vi "Test.vi"() -> ()   [LabVIEW 2018]
uses:
  utils/Return_t.ctl
  <vilib>/Instr/_visa.llb/VISA Configure Serial Port (Instr).vi
panel:
  out "Read DATA Str":string
  out "Str EPC":string
  out "EPC Bytes":u8
  out "Freq (Mhz)":dbl
  out "RSSI":i32
  out "Return":T1
  out "Shift Data":u16
  out "Msg Length":u16
  out "FF?":bool
  in  "stop":bool
  in  "Test":bool
  in  "Power":u32=500 max=2700 step=10
  out "error out":errorcluster
  out "Read DATA HEX":string
  in  "Delay":u16=1200
  out "Set Err":errorcluster
  out "WR Str":string
  out "Ini ?":bool
  in  "COM RFID":refnum<visa-resource-name>="COM4"
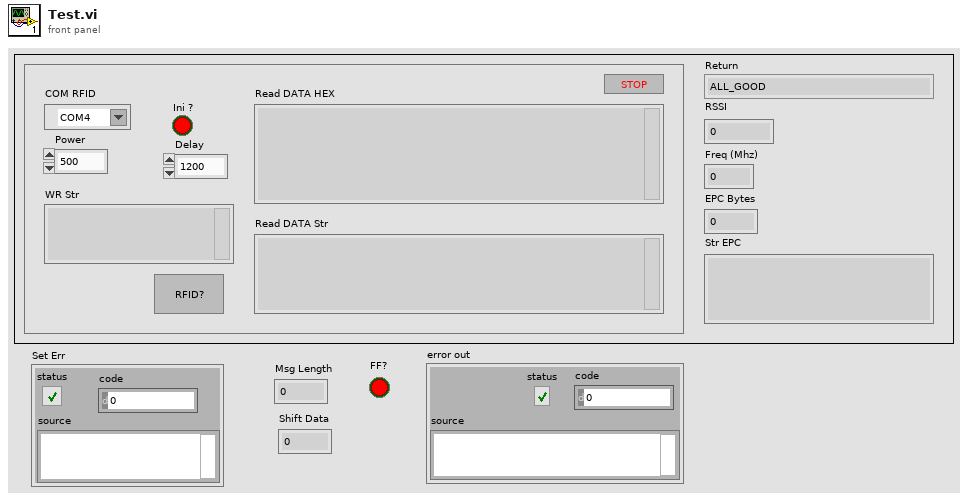
[diagram p1: front panel]
types:
  T1 = typedef "Return_t.ctl" = enum16{"ALL_GOOD", "ERROR_COMMAND_RESPONSE_TIMEOUT", "ERROR_CORRUPT_RESPONSE", "ERROR_WRONG_OPCODE_RESPONSE", "ERROR_UNKNOWN_OPCODE", "RESPONSE_IS_TEMPERATURE", "RESPONSE_IS_KEEPALIVE", "RESPONSE_IS_TEMPTHROTTLE", "RESPONSE_IS_TAGFOUND", "RESPONSE_IS_NOTAGFOUND", "RESPONSE_IS_UNKNOWN", "RESPONSE_SUCCESS", "RESPONSE_FAIL"}
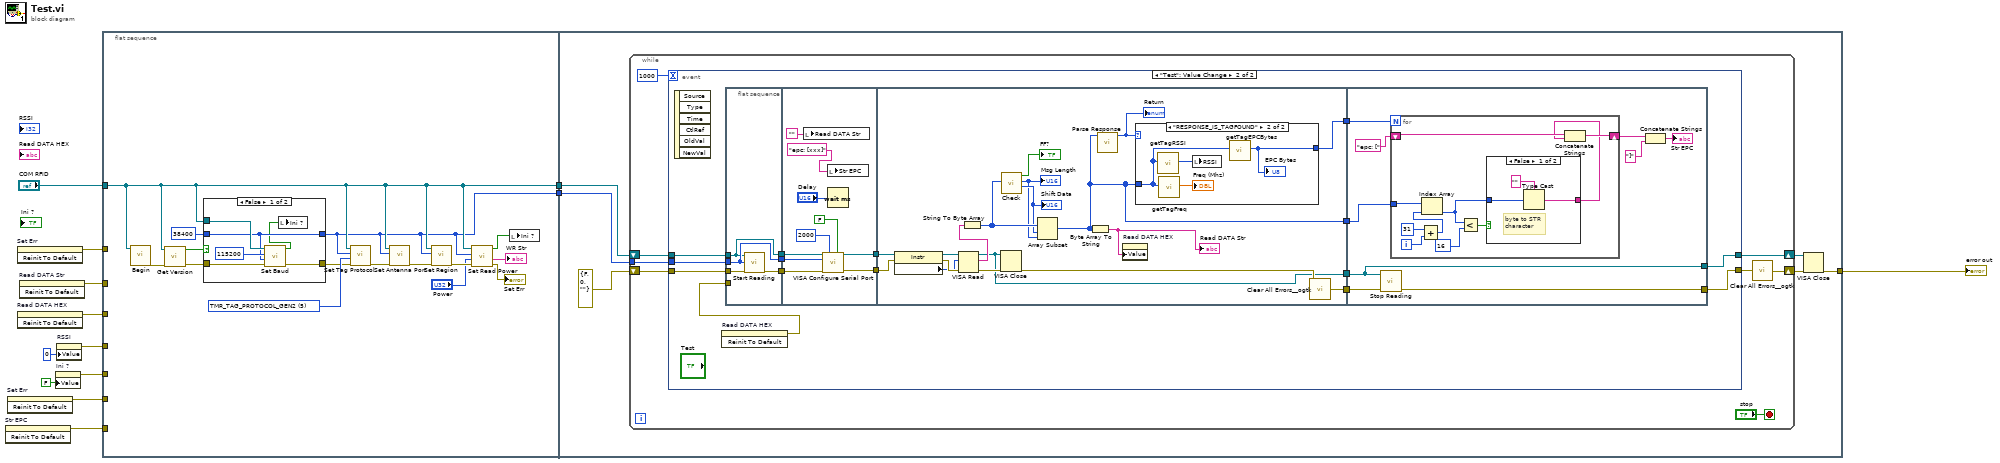
[diagram p0: block diagram]
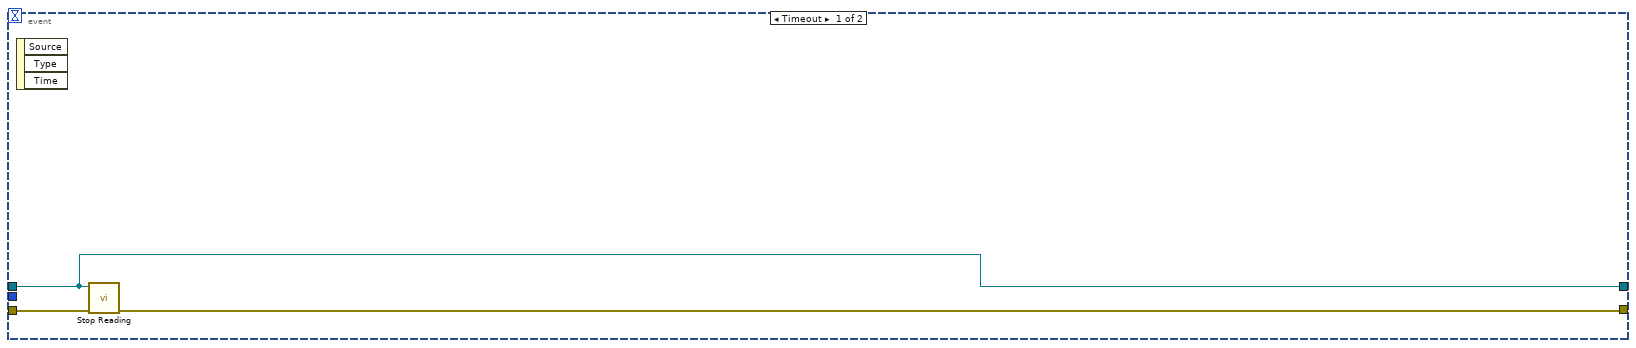
[diagram p3: hidden frame]
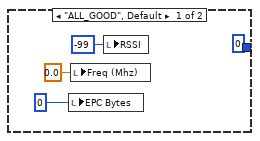
[diagram p4: hidden frame]
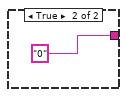
[diagram p5: hidden frame]
diagram:
  n1 = invoke on="Str EPC" class="Str" method="Reinit To Default"() -> (error out=w1:errorcluster)  [unwired: 3 in, 2 out]
  n2 = invoke on="Set Err" class="Clust (strict)" method="Reinit To Default"() -> (error out=w3:errorcluster)  [unwired: 3 in, 2 out]
  n3 = invoke on="Set Err" class="Clust (strict)" method="Reinit To Default"() -> (error out=w11:errorcluster)  [unwired: 3 in, 2 out]
  n4 = invoke on="Read DATA HEX" class="Str" method="Reinit To Default"() -> (error out=w10:errorcluster)  [unwired: 3 in, 2 out]
  n5 = invoke on="Read DATA Str" class="Str" method="Reinit To Default"() -> (error out=w2:errorcluster)  [unwired: 3 in, 2 out]
  n6 = property on="Ini ?" class="Bool (strict)"("Value"=FALSE ("Ini ?")) -> (error out=w4:errorcluster)  [unwired: 2 in, 1 out]
  n7 = property on="RSSI" class="DigNum (strict)"("Value"=u8 0 ("RSSI")) -> (error out=w7:errorcluster)  [unwired: 2 in, 1 out]
  n8 = flat-sequence {
    tunnel: [w28] -> w12
    tunnel: [w27] -> w8
    tunnel: w7 -> [_]
    tunnel: w10 -> [_]
    tunnel: w11 -> [_]
    tunnel: "COM RFID" -> [w28]
    tunnel: w4 -> [_]
    tunnel: w3 -> [_]
    tunnel: w2 -> [_]
    tunnel: w1 -> [_]
    tunnel: w12 -> [w38]
    tunnel: [w40] -> w9
    tunnel: w8 -> [w37]
    frame #0 {
      w26 = u16 5 items=["TMR_TAG_PROTOCOL_NONE"=0, "TMR_TAG_PROTOCOL_ISO180006B"=3, "TMR_TAG_PROTOCOL_GEN2"=5, "TMR_TAG_PROTOCOL_ISO180006B_UCODE"=6, "TMR_TAG_PROTOCOL_IPX64"=7, "TMR_TAG_PROTOCOL_IPX256"=8, "TMR_TAG_PROTOCOL_ATA"=29] ("Tag Protocol")
      n9 = call "Begin.vi"("COM Port"=w28) -> ("error out"=w18:errorcluster)  [unwired: 10 in]
      n10 = call "Get Version.vi"("error in (no error)"=w18, "COM Port"=w28) -> ("error out"=w17:errorcluster, "Result"=w16:bool)  [unwired: 7 in, 1 out]
      n11 = case shown="False" w16 {
        tunnel: [w33 w36] -> w19
        tunnel: [w30 w35] -> w27
        tunnel: w17 -> [w32 w36]
        tunnel: w28 -> [w31 _]
        tunnel: u32 38400 ("New Baud") -> [w30 w35]
        frame False {
          n12 = call "Set Baud.vi"("error in (no error)"=w32, "New Baud"=w30, "Old Baud"=u32 115200, "COM Port"=w31) -> ("error out"=w33:errorcluster, "Result"=w29:bool)  [unwired: 6 in]
          n13 = local write "Ini ?"(w29) -> ()
        }
        frame True {
        }
      }
      n14 = call "Set Tag Protocol.vi"("error in (no error)"=w19, "Protocol"=w26, "Baud Rate"=w27, "COM Port"=w28) -> ("error out"=w25:errorcluster)  [unwired: 5 in, 2 out]
      n15 = call "Set Antenna Port.vi"("error in (no error)"=w25, "Baud Rate"=w27, "COM Port"=w28) -> ("error out"=w24:errorcluster)  [unwired: 6 in, 2 out]
      n16 = call "Set Region.vi"("error in (no error)"=w24, "Baud Rate"=w27, "COM Port"=w28) -> ("error out"=w23:errorcluster)  [unwired: 6 in, 2 out]
      n17 = call "Set Read Power.vi"("error in (no error)"=w23, "Power"="Power", "Baud"=w27, "COM Port"=w28) -> ("error out"=→"Set Err":errorcluster, "received str"=→"WR Str":string, "Result"=w14:bool)  [unwired: 5 in]
      n18 = local write "Ini ?"(w14) -> ()
    }
    frame #1 {
      n19 = while {
        shift-right: [w44] -> w42
        shift-left: w38 -> [w49]
        shift-right: [w46] -> w41
        shift-left: errorcluster {"status"=FALSE, "code"=0, "source"=""} ("error out") -> [w48]
        tunnel: w37 -> [w43]
        stop <- "stop" stop-if-true
        n20 = event shown="[1] \"Test\": Value Change" {
          selector: _ -> [_ _]
          dyn-events: _ -> [_ _]
          timeout: 1000 -> [_ _]
          tunnel: w49 -> [w52 w68]
          tunnel: w48 -> [w53 w67]
          tunnel: [w52 w60] -> w44
          tunnel: [w51 w61] -> w45
          tunnel: w43 -> [_ w66]
          event Timeout {
            n21 = event-data() -> ()  [unwired: 1 in, 3 out]
            n22 = call "Stop Reading.vi"("error in (no error)"=w53, "COM Port"=w52) -> ("error out"=w51:errorcluster)  [unwired: 7 in, 2 out]
          }
          event "Test": Value Change {
            n23 = event-data() -> ()  [unwired: 1 in, 6 out]
            n24 = invoke on="Read DATA HEX" class="Str" method="Reinit To Default"() -> (error out=w56:errorcluster)  [unwired: 3 in, 2 out]
            n25 = flat-sequence {
              tunnel: w68 -> [w69]
              tunnel: w67 -> [w72]
              tunnel: w66 -> [w70]
              tunnel: [w71] -> w65
              tunnel: [w70] -> w64
              tunnel: [w69] -> w62
              tunnel: w56 -> [_]
              tunnel: w65 -> [w78]
              tunnel: w64 -> [w77]
              tunnel: w62 -> [w79]
              tunnel: [w81] -> w59
              tunnel: [w80] -> w58
              tunnel: [w87] -> w63
              tunnel: w59 -> [w100]
              tunnel: w58 -> [w99]
              tunnel: [w90] -> w57
              tunnel: [w86] -> w55
              tunnel: [w85] -> w54
              tunnel: w63 -> [w115]
              tunnel: [w116] -> w61
              tunnel: [w115] -> w60
              tunnel: w57 -> [w117]
              tunnel: w55 -> [w114]
              tunnel: w54 -> [w111]
              frame #0 {
                n26 = call "Start Reading.vi"("error in (no error)"=w72, "Baud Rate"=w70, "COM Port"=w69) -> ("error out"=w71:errorcluster)  [unwired: 6 in, 2 out]
              }
              frame #1 {
                n27 = local write "Read DATA Str"("") -> ()
                n28 = call-poly "VISA Configure Serial Port"("VISA resource name"=w79, "timeout (10sec)"=u32 2000, "Enable Termination\nChar (T)"=FALSE ("Enable Termination\nChar (T)"), "baud rate (9600)"=w77, "error in (no error)"=w78) -> ("VISA resource name out"=w81:refnum<visa-resource-name>, "error out"=w80:errorcluster)  [unwired: 9 in]
                n29 = local write "Str EPC"("epc: [xxx]") -> ()
                n30 = Wait (ms)(milliseconds to wait="Delay") -> ()  [unwired: 1 out]
              }
              frame #2 {
                n31 = property class="Instr"(reference=w100, error in=w99) -> (reference out=w96:refnum<visa-resource-name>, error out=w98:errorcluster, "Serial Settings:Number of Bytes at Serial Port"=w97:u32)
                n32 = VISA Read(VISA resource name=w96, byte count=w97, error in (no error)=w98) -> (VISA resource name out=w87:refnum<visa-resource-name>, read buffer=w88:string, error out=w91:errorcluster)  [unwired: 1 out]
                n33 = String To Byte Array(string=w88) -> (unsigned byte array=w95:u8[])
                n34 = VISA Close(VISA resource name=w87, error in (no error)=w91) -> (error out=w89:errorcluster)
                n35 = call "Check.vi"("Date"=w95) -> ("Shift Data"=w93:u16, "Msg Length"=w92:u16, "Result"=→"FF?":bool)  [unwired: 8 in]
                "Msg Length" <- w92
                "Shift Data" <- w93
                n36 = Array Subset(array=w95, index=w93, length=w92) -> (w85:u8[])
                n37 = Byte Array To String(unsigned byte array=w85) -> (string=w83:string)
                "Read DATA Str" <- w83
                n38 = call "Parse Response.vi"("Data Array"=w85) -> ("Return"=w84:T1)  [unwired: 10 in]
                "Return" <- w84
                n39 = property on="Read DATA HEX" class="Str"("Value"=w83) -> ()  [unwired: 2 in, 2 out]
                n40 = case shown="\"RESPONSE_IS_TAGFOUND\"" w84 {
                  tunnel: w85 -> [_ w106]
                  tunnel: [u8 0 ("EPC Bytes") w105] -> w86
                  frame "ALL_GOOD", Default {
                    n41 = local write "EPC Bytes"(u8 0 ("Butes Cnt")) -> ()
                    n42 = local write "Freq (Mhz)"(0.0 ("Freq (Mhz)")) -> ()
                    n43 = local write "RSSI"(-99 ("RSSI")) -> ()
                  }
                  frame "RESPONSE_IS_TAGFOUND" {
                    n44 = call "getTagRSSI.vi"("Data Arry"=w106) -> ("RSSI"=w108:i32)  [unwired: 10 in]
                    n45 = call "getTagFreq.vi"("Data Array"=w106) -> ("Freq"=→"Freq (Mhz)":dbl)  [unwired: 10 in]
                    n46 = local write "RSSI"(w108) -> ()
                    n47 = call "getTagEPCBytes.vi"("Data Arry"=w106) -> ("EPC Bytes"=w105:u8)  [unwired: 10 in]
                    "EPC Bytes" <- w105
                  }
                }
                n48 = call <userlib>:"Clear All Errors__ogtk.vi"("Error In"=w89) -> ("Error Out"=w90:errorcluster)  [unwired: 3 in]
              }
              frame #3 {
                n49 = call "Stop Reading.vi"("error in (no error)"=w117, "COM Port"=w115) -> ("error out"=w116:errorcluster)  [unwired: 7 in, 2 out]
                n50 = for {
                  N: w114 -> [_]
                  shift-right: [w126] -> w110
                  shift-left: "epc: [" -> [w127]
                  tunnel: w111 -> [w122]
                  i -> [w125]
                  n51 = Add(x=31, y=w125) -> (x+y=w123:i32)
                  n52 = Index Array(array=w122, index=w123) -> (element=w119:u8)
                  n53 = Less?(x=w119, y=u8 16) -> (x < y?=w120:bool)
                  n54 = case shown="False" w120 {
                    tunnel: w119 -> [w130 _]
                    tunnel: [w129 "0"] -> w118
                    frame False {
                      # "byte to STR\ncharacter"
                      n55 = Type Cast(type="", x=w130) -> (*(type *) &x=w129:string)
                    }
                    frame True {
                    }
                  }
                  n56 = Concatenate Strings(w127, w118) -> (w126:string)
                }
                n57 = Concatenate Strings(w110, "]" ("string")) -> (→"Str EPC":string)
              }
            }
          }
        }
        n58 = call <userlib>:"Clear All Errors__ogtk.vi"("Error In"=w45) -> ("Error Out"=w46:errorcluster)  [unwired: 3 in]
      }
      n59 = VISA Close(VISA resource name=w42, error in (no error)=w41) -> (error out=w40:errorcluster)
    }
  }
  "error out" <- w9
